vi "Get CAN Port List.vi"() -> (3 "CAN Port List":string[](array[string]))   [LabVIEW 2021, in "Performanced XNET CAN Signal Logger.lvlib" / "Performanced XNET CAN Signal Logger.lvclass"]
uses:
  Performanced XNET CAN Signal Logger.lvclass
  <vilib>/nisyscfg/Close (System).vi
  Performanced XNET CAN Signal Logger.lvclass/Performanced XNET CAN Signal Logger.ctl
  <vilib>/nisyscfg/nisyscfg.lvlib
  <resource>/objmgr/nisysapi.rc
  <resource>/objmgr/nicontrollersysapi.rc
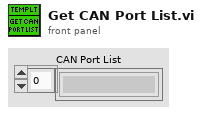
[diagram p1: front panel]
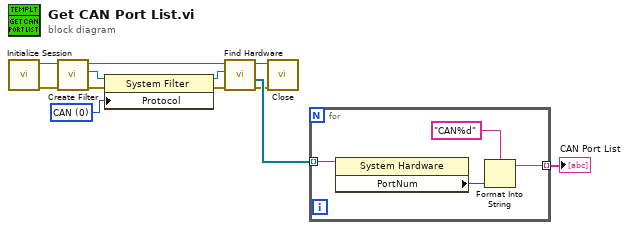
[diagram p0: block diagram]
diagram:
  w9 = u32 0 items=["CAN"=0, "FlexRay"=1, "LIN"=2, "Ethernet"=3, "Unknown"=4294967294] ("XNET:Interface:Protocol")
  n1 = call <vilib>:"Initialize Session.vi"() -> ("error out"=w4:errorcluster, "Session out"=w6:refnum<k21>)  [unwired: 10 in]
  n2 = call <vilib>:"Create Filter.vi"("error in (no error)"=w4, "Session in"=w6) -> ("error out"=w12:errorcluster, "Filter out"=w11:refnum<k20>, "Session out"=w5:refnum<k21>)  [unwired: 7 in]
  n3 = property class="System Filter"(reference=w11, error in=w12, "Protocol"=w9) -> (reference out=w10:refnum<k20>, error out=w3:errorcluster)
  n4 = call <vilib>:"Find Hardware.vi"("error in (no error)"=w3, "Filter in"=w10, "Session in"=w5) -> ("error out"=w2:errorcluster, "Resources out"=w7:refnum<k20>[], "Session out"=w8:refnum<k21>)  [unwired: 5 in, 1 out]
  n5 = call-poly <vilib>:"Close.vi"("error in (no error)"=w2, "Session in"=w8) -> ()  [unwired: 9 in, 1 out]
  n6 = for {
    tunnel: w7 -> [w16] mode=indexing
    tunnel: [w13] -> w1 mode=indexing
    n7 = property class="System Hardware"(reference=w16) -> ("PortNum"=w15:u32)  [unwired: 1 in, 2 out]
    n8 = Format Into String(format string="CAN%d", w15) -> (resulting string=w13:string)  [unwired: 2 in, 1 out]
  }
  "CAN Port List" <- w1
